vi "PC Engine.vi"(2 "Error In":errorcluster) -> (0 "Error Out":errorcluster, 1 "InvalidResponses":string)   [LabVIEW 2013]
uses:
  State Ctrl (PC).ctl
  <vilib>/NI/STM/TCP/TCP Connection Info.ctl
  <vilib>/NI/STM/SubVIs/MetaDataElement.ctl
  Event Mode.ctl
  <vilib>/NI/STM/TCP/TCP Read Options.ctl
  RT/RTsend PCrecv CMD.ctl
  TypeDef/ConnSettingCluster.ctl
  <vilib>/NI/STM/TCP/Read Meta Data (TCP Ref).vi
  <vilib>/NI/STM/TCP/Read Message (TCP).vi
  <vilib>/NI/STM/TCP/Read Meta Data (TCP Clst).vi
  <vilib>/NI/STM/TCP/Write Message (TCP).vi
  <vilib>/NI/STM/NI STM.lvlib
panel:
  out "Send Conn Info":T1
  in  "State Control":T3
  in  "Recv Port":u16=5555
  in  "Stop":bool
  out "Connected?":bool
  in  "ConnectAttemptLimit":u32=5
  in  "Send Port":u16=5555
  in  "RIO IP Address":string
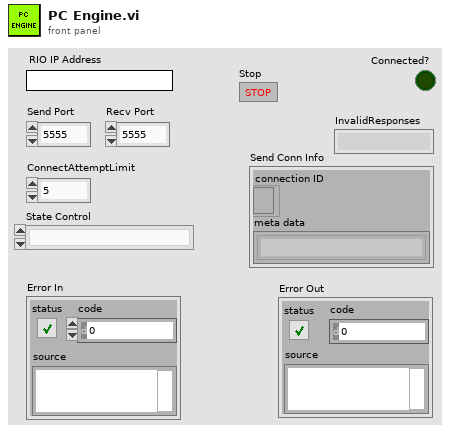
[diagram p1: front panel]
types:
  T1 = typedef "NI STM.lvlib/TCP Connection Info.ctl" = cluster{"connection ID":refnum<k5>, "meta data":T2[]}
  T2 = typedef "NI STM.lvlib/MetaDataElement.ctl" = string
  T3 = typedef "State Ctrl (PC).ctl" = enum16{"", "Send Connect", "Send Connect 2", "Recv Connect", "Recv Connect 2", "No Connection", "Disconnect"}
  T4 = typedef "Event Mode.ctl" = enum16{"Init", "Get", "Set", "Destroy"}
  T5 = cluster{"Command":string, "Flattened Data":string}
  T6 = typedef "PCsend RTrecv CMD.ctl" = enum16{"ConnSettings", "Connect", "Stop", "Digital Outputs", "Analog Outputs", "Sweep Parameters", "Start Sweep", "Cal2RT", "Save Cal", "Load Cal"}
  T7 = typedef "ConnSettingCluster.ctl" = cluster{"ConnectAttemptLimit(5)":u32, "IP Address":string, "Send Port":u16, "Recv Port":u16}
  T8 = typedef "NI STM.lvlib/TCP Read Options.ctl" = cluster{"ignore timeout error":bool, "timeout ms (1000)":i32}
  T9 = typedef "RTsend PCrecv CMD.ctl" = enum16{"Digital Inputs", "Connected?", "Data", "Data 2", "Cal2PC"}
  T10 = cluster{"connection ID":bool, "meta data":bool[]}
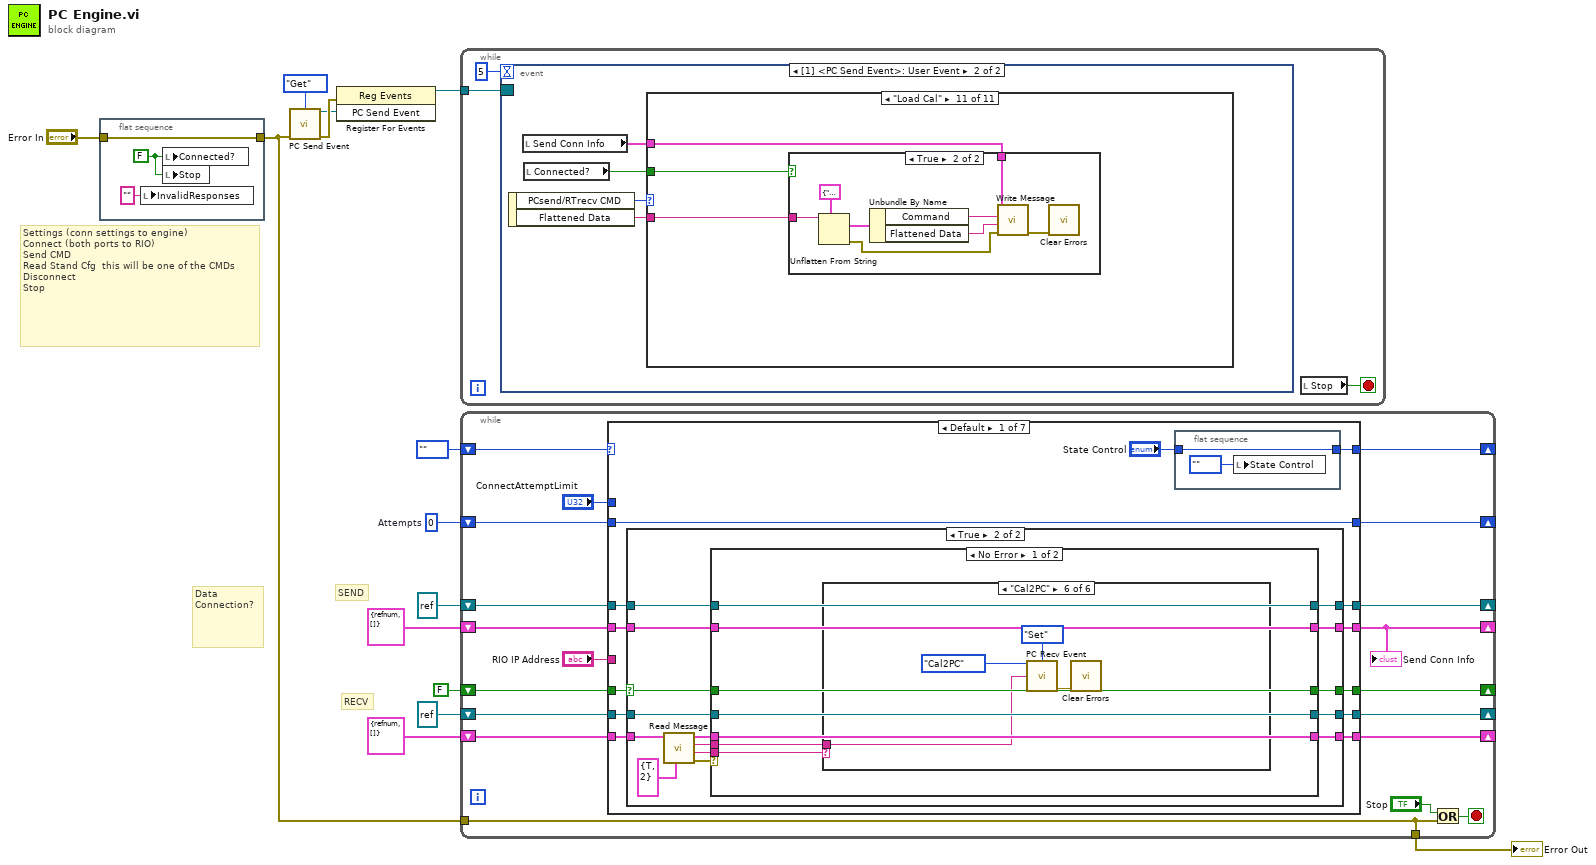
[diagram p0: block diagram]
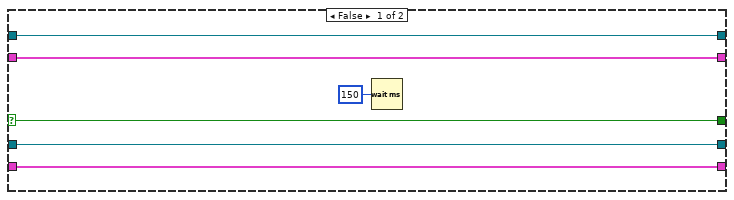
[diagram p2: hidden frame]
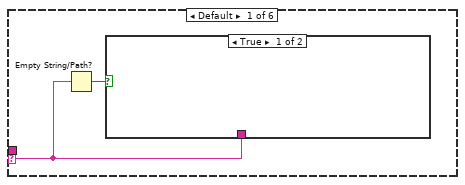
[diagram p3: hidden frame]
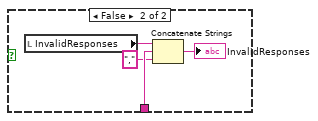
[diagram p4: hidden frame]
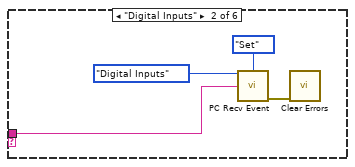
[diagram p5: hidden frame]
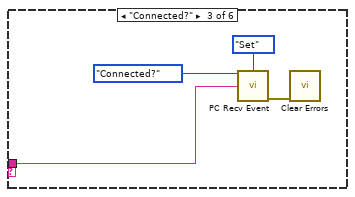
[diagram p6: hidden frame]
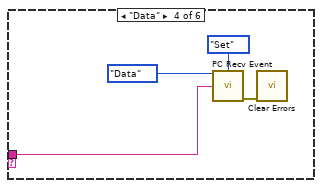
[diagram p7: hidden frame]
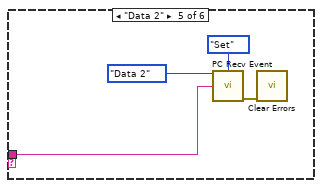
[diagram p8: hidden frame]
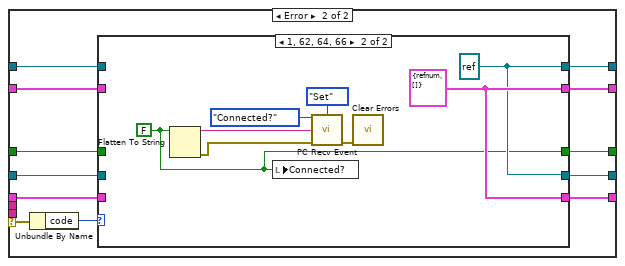
[diagram p9: hidden frame]
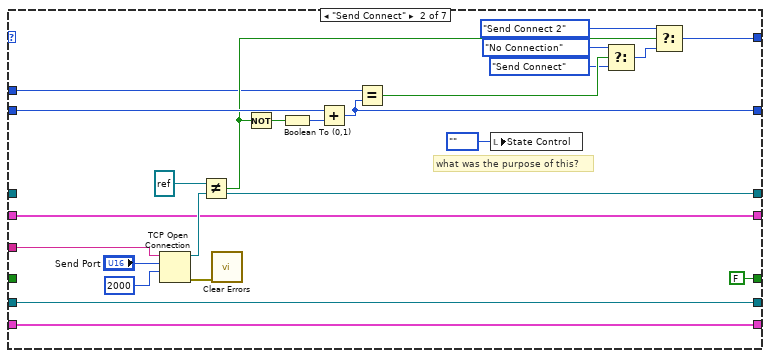
[diagram p11: hidden frame]
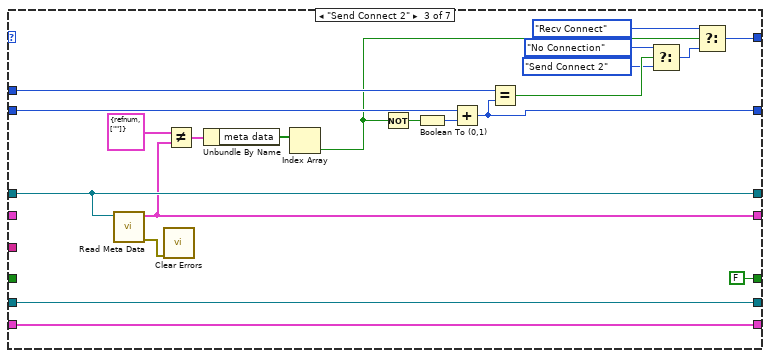
[diagram p12: hidden frame]
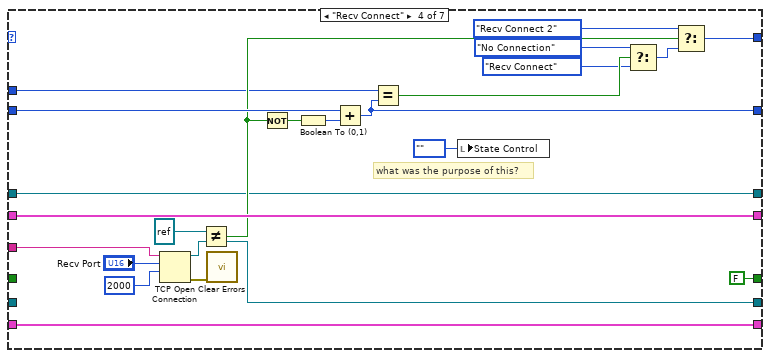
[diagram p13: hidden frame]
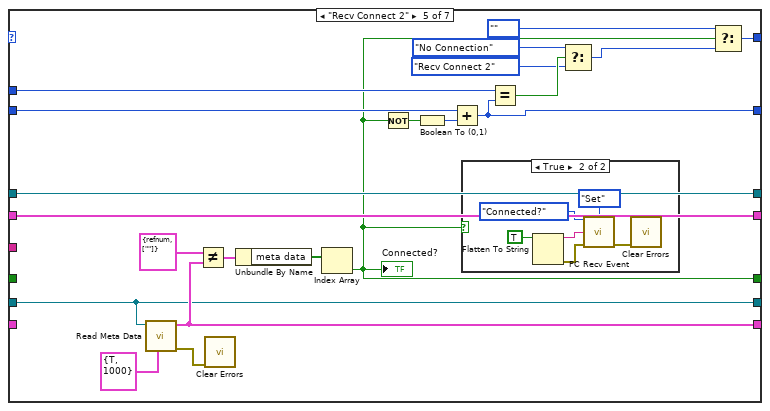
[diagram p14: hidden frame]
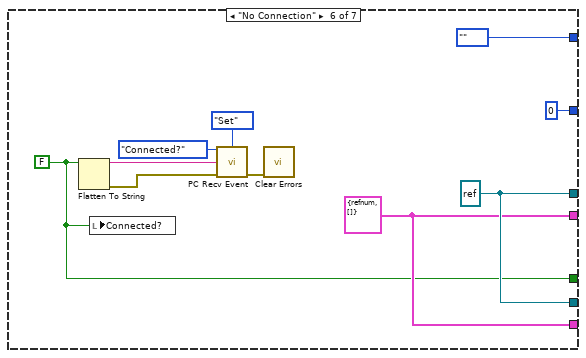
[diagram p16: hidden frame]
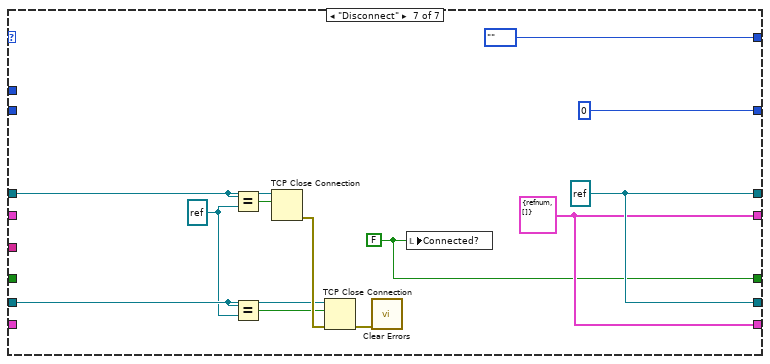
[diagram p17: hidden frame]
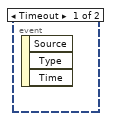
[diagram p18: hidden frame]
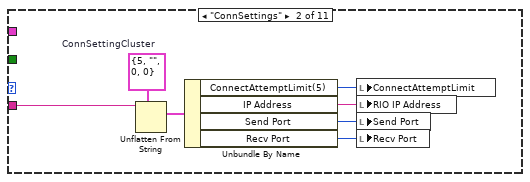
[diagram p20: hidden frame]
diagram:
  w12 = u32 0  # Attempts
  # "RECV"
  # "SEND"
  # "Data\nConnection?"
  # "Settings (conn settings to engine)\nConnect (both ports to RIO)\nSend CMD\nRead Stand Cfg  this will be one of the CMDs\nDisconnect\nStop"
  n1 = flat-sequence {
    tunnel: "Error In" -> [w16]
    tunnel: [w16] -> w10
    frame #0 {
      w17 = FALSE ("Connected?")
      n2 = local write "InvalidResponses"("" ("InvalidResponse")) -> ()
      n3 = local write "Connected?"(w17) -> ()
      n4 = local write "Stop"(w17) -> ()
    }
  }
  n5 = call "PC Send Event.vi"("Mode"=Event_Mode."Get", "Error In"=w10) -> ("PC Send Event"=w5:refnum<user-event>, "Error Out"=w7:errorcluster)  [unwired: 12 in]
  n6 = register-events(error in=w7, w5) -> (reference out=w6:refnum<event-registration>)  [unwired: 1 in, 1 out]
  n7 = while {
    tunnel: w6 -> [w18]
    stop <- w20 stop-if-true
    n8 = event shown="[1] <PC Send Event>: User Event" {
      selector: w18 -> [_ _]
      dyn-events: _ -> [_ _]
      timeout: 5 ("evtime") -> [_ _]
      event Timeout {
        n9 = event-data() -> ()  [unwired: 1 in, 3 out]
      }
      event User Event {
        n10 = event-data() -> ("PCsend/RTrecv CMD"=w21:T6, "Flattened Data"=w24:string)  [unwired: 1 in]
        n11 = local read "Send Conn Info"() -> (w23:T1)
        n12 = local read "Connected?"() -> (w22:bool)
        n13 = case shown="\"Load Cal\"" w21 {
          tunnel: w24 -> [_ w26 _ w36 w47 w58 w69 w80 w91 w102 w113]
          tunnel: w23 -> [_ _ _ w34 w45 w56 w67 w78 w89 w100 w111]
          tunnel: w22 -> [_ _ _ w35 w46 w57 w68 w79 w90 w101 w112]
          frame Default {
          }
          frame "ConnSettings" {
            w25 = T7 {"ConnectAttemptLimit(5)"=5, "IP Address"="", "Send Port"=0, "Recv Port"=0}  # ConnSettingCluster
            n14 = Unflatten From String(type=w25, binary string=w26) -> (value=w31:T7)  [unwired: 3 in, 2 out]
            n15 = Unbundle By Name(w31) -> ("ConnectAttemptLimit(5)"=w29:u32, "IP Address"=w28:string, "Send Port"=w30:u16, "Recv Port"=w27:u16)
            n16 = local write "ConnectAttemptLimit"(w29) -> ()
            n17 = local write "RIO IP Address"(w28) -> ()
            n18 = local write "Send Port"(w30) -> ()
            n19 = local write "Recv Port"(w27) -> ()
          }
          frame "Connect" {
            n20 = local write "State Control"(State_Ctrl_(PC)."Send Connect" ("State Control")) -> ()
          }
          frame "Stop" {
            n21 = case shown="True" w35 {
              tunnel: w36 -> [_ w44]
              tunnel: w34 -> [_ w39]
              frame False {
              }
              frame True {
                n22 = Unflatten From String(type=T5 {"Command"="", "Flattened Data"=""} ("cluster"), binary string=w44) -> (value=w43:T5, error out=w37:errorcluster)  [unwired: 3 in, 1 out]
                n23 = Unbundle By Name(w43) -> ("Command"=w40:string, "Flattened Data"=w41:string)
                n24 = call-poly <vilib>:"Write Message.vi"("error in"=w37, "data"=w41, "name"=w40, "connection info in"=w39) -> ("error out"=w38:errorcluster)  [unwired: 6 in, 1 out]
                n25 = call <vilib>:"Clear Errors.vi"("error in (no error)"=w38) -> ()  [unwired: 6 in, 1 out]
              }
            }
            n26 = local write "Stop"(TRUE ("Stop")) -> ()
          }
          frame "Digital Outputs" {
            n27 = case shown="False" w46 {
              tunnel: w47 -> [_ w55]
              tunnel: w45 -> [_ w50]
              frame False {
              }
              frame True {
                n28 = Unflatten From String(type=T5 {"Command"="", "Flattened Data"=""} ("cluster"), binary string=w55) -> (value=w54:T5, error out=w48:errorcluster)  [unwired: 3 in, 1 out]
                n29 = Unbundle By Name(w54) -> ("Command"=w51:string, "Flattened Data"=w52:string)
                n30 = call-poly <vilib>:"Write Message.vi"("error in"=w48, "data"=w52, "name"=w51, "connection info in"=w50) -> ("error out"=w49:errorcluster)  [unwired: 6 in, 1 out]
                n31 = call <vilib>:"Clear Errors.vi"("error in (no error)"=w49) -> ()  [unwired: 6 in, 1 out]
              }
            }
          }
          frame "Analog Outputs" {
            n32 = case shown="True" w57 {
              tunnel: w58 -> [_ w66]
              tunnel: w56 -> [_ w61]
              frame False {
              }
              frame True {
                n33 = Unflatten From String(type=T5 {"Command"="", "Flattened Data"=""} ("cluster"), binary string=w66) -> (value=w65:T5, error out=w59:errorcluster)  [unwired: 3 in, 1 out]
                n34 = Unbundle By Name(w65) -> ("Command"=w62:string, "Flattened Data"=w63:string)
                n35 = call-poly <vilib>:"Write Message.vi"("error in"=w59, "data"=w63, "name"=w62, "connection info in"=w61) -> ("error out"=w60:errorcluster)  [unwired: 6 in, 1 out]
                n36 = call <vilib>:"Clear Errors.vi"("error in (no error)"=w60) -> ()  [unwired: 6 in, 1 out]
              }
            }
          }
          frame "Sweep Parameters" {
            n37 = case shown="True" w68 {
              tunnel: w69 -> [_ w77]
              tunnel: w67 -> [_ w72]
              frame False {
              }
              frame True {
                n38 = Unflatten From String(type=T5 {"Command"="", "Flattened Data"=""} ("cluster"), binary string=w77) -> (value=w76:T5, error out=w70:errorcluster)  [unwired: 3 in, 1 out]
                n39 = Unbundle By Name(w76) -> ("Command"=w73:string, "Flattened Data"=w74:string)
                n40 = call-poly <vilib>:"Write Message.vi"("error in"=w70, "data"=w74, "name"=w73, "connection info in"=w72) -> ("error out"=w71:errorcluster)  [unwired: 6 in, 1 out]
                n41 = call <vilib>:"Clear Errors.vi"("error in (no error)"=w71) -> ()  [unwired: 6 in, 1 out]
              }
            }
          }
          frame "Start Sweep" {
            n42 = case shown="True" w79 {
              tunnel: w80 -> [_ w88]
              tunnel: w78 -> [_ w83]
              frame False {
              }
              frame True {
                n43 = Unflatten From String(type=T5 {"Command"="", "Flattened Data"=""} ("cluster"), binary string=w88) -> (value=w87:T5, error out=w81:errorcluster)  [unwired: 3 in, 1 out]
                n44 = Unbundle By Name(w87) -> ("Command"=w84:string, "Flattened Data"=w85:string)
                n45 = call-poly <vilib>:"Write Message.vi"("error in"=w81, "data"=w85, "name"=w84, "connection info in"=w83) -> ("error out"=w82:errorcluster)  [unwired: 6 in, 1 out]
                n46 = call <vilib>:"Clear Errors.vi"("error in (no error)"=w82) -> ()  [unwired: 6 in, 1 out]
              }
            }
          }
          frame "Cal2RT" {
            n47 = case shown="True" w90 {
              tunnel: w91 -> [_ w99]
              tunnel: w89 -> [_ w94]
              frame False {
              }
              frame True {
                n48 = Unflatten From String(type=T5 {"Command"="", "Flattened Data"=""} ("cluster"), binary string=w99) -> (value=w98:T5, error out=w92:errorcluster)  [unwired: 3 in, 1 out]
                n49 = Unbundle By Name(w98) -> ("Command"=w95:string, "Flattened Data"=w96:string)
                n50 = call-poly <vilib>:"Write Message.vi"("error in"=w92, "data"=w96, "name"=w95, "connection info in"=w94) -> ("error out"=w93:errorcluster)  [unwired: 6 in, 1 out]
                n51 = call <vilib>:"Clear Errors.vi"("error in (no error)"=w93) -> ()  [unwired: 6 in, 1 out]
              }
            }
          }
          frame "Save Cal" {
            n52 = case shown="True" w101 {
              tunnel: w102 -> [_ w110]
              tunnel: w100 -> [_ w105]
              frame False {
              }
              frame True {
                n53 = Unflatten From String(type=T5 {"Command"="", "Flattened Data"=""} ("cluster"), binary string=w110) -> (value=w109:T5, error out=w103:errorcluster)  [unwired: 3 in, 1 out]
                n54 = Unbundle By Name(w109) -> ("Command"=w106:string, "Flattened Data"=w107:string)
                n55 = call-poly <vilib>:"Write Message.vi"("error in"=w103, "data"=w107, "name"=w106, "connection info in"=w105) -> ("error out"=w104:errorcluster)  [unwired: 6 in, 1 out]
                n56 = call <vilib>:"Clear Errors.vi"("error in (no error)"=w104) -> ()  [unwired: 6 in, 1 out]
              }
            }
          }
          frame "Load Cal" {
            n57 = case shown="True" w112 {
              tunnel: w113 -> [_ w121]
              tunnel: w111 -> [_ w116]
              frame False {
              }
              frame True {
                n58 = Unflatten From String(type=T5 {"Command"="", "Flattened Data"=""} ("cluster"), binary string=w121) -> (value=w120:T5, error out=w114:errorcluster)  [unwired: 3 in, 1 out]
                n59 = Unbundle By Name(w120) -> ("Command"=w117:string, "Flattened Data"=w118:string)
                n60 = call-poly <vilib>:"Write Message.vi"("error in"=w114, "data"=w118, "name"=w117, "connection info in"=w116) -> ("error out"=w115:errorcluster)  [unwired: 6 in, 1 out]
                n61 = call <vilib>:"Clear Errors.vi"("error in (no error)"=w115) -> ()  [unwired: 6 in, 1 out]
              }
            }
          }
        }
      }
    }
    n62 = local read "Stop"() -> (w20:bool)
  }
  n63 = while {
    shift-right: [w135] -> _
    shift-left: refnum<k5> refnum ("connection ID") -> [w138]
    shift-right: [w136] -> _
    shift-left: T1 {"connection ID"=refnum, "meta data"=[]} ("connection info out") -> [w137]
    shift-right: [w139] -> _
    shift-left: State_Ctrl_(PC)."" ("State Control") -> [w140]
    shift-right: [w133] -> _
    shift-left: w12 -> [w134]
    tunnel: w10 -> [w122]
    shift-right: [w126] -> _
    shift-left: refnum<k5> refnum ("connection ID") -> [w128]
    shift-right: [w125] -> _
    shift-left: T1 {"connection ID"=refnum, "meta data"=[]} ("connection info out") -> [w127]
    shift-right: [w123] -> _
    shift-left: FALSE -> [w124]
    tunnel: [w122] -> w1
    stop <- w131 stop-if-true
    n64 = case shown="Default" w140 {
      tunnel: [w153 w257 w275 w301 w319 State_Ctrl_(PC)."" ("State Control") State_Ctrl_(PC)."" ("State Control")] -> w139
      tunnel: w138 -> [w148 _ w276 w283 w320 _ w345]
      tunnel: w137 -> [w149 w252 _ w298 w307 _ _]
      tunnel: [w145 w252 w259 w298 w307 w333 w347] -> w136
      tunnel: [w146 w253 w276 w283 w320 w334 w348] -> w135
      tunnel: w134 -> [w141 w251 w271 w297 w315 _ _]
      tunnel: [w141 w247 w270 w293 w314 u32 0 ("Attempts") u32 0 ("Attempts")] -> w133
      tunnel: "ConnectAttemptLimit" -> [_ w244 w268 w290 w312 _ _]
      tunnel: "RIO IP Address" -> [_ w239 _ w285 _ _ _]
      tunnel: w128 -> [w147 w238 w264 _ w306 _ w342]
      tunnel: w127 -> [w150 w237 w263 w281 _ _ _]
      tunnel: [w143 w238 w264 w282 w306 w334 w348] -> w126
      tunnel: [w142 w237 w263 w281 w308 w333 w347] -> w125
      tunnel: w124 -> [w151 _ _ _ _ _ _]
      tunnel: [w144 FALSE ("Meta Element") FALSE ("Meta Element") FALSE ("Meta Element") w303 w332 w340] -> w123
      frame Default {
        n65 = case shown="True" w151 {
          selector: w151 -> [w157 w168]
          tunnel: w150 -> [w155 w173]
          tunnel: w149 -> [w158 w169]
          tunnel: w148 -> [w159 w167]
          tunnel: w147 -> [w156 w170]
          tunnel: [w159 w165] -> w146
          tunnel: [w158 w163] -> w145
          tunnel: [w157 w166] -> w144
          tunnel: [w156 w164] -> w143
          tunnel: [w155 w162] -> w142
          frame False {
            n66 = Wait (ms)(milliseconds to wait=u32 150) -> ()  [unwired: 1 out]
          }
          frame True {
            n67 = call-poly <vilib>:"Read Message.vi"("options"=T8 {"ignore timeout error"=TRUE, "timeout ms (1000)"=2}, "connection info in"=w173) -> ("error out"=w172:errorcluster, "name"=w161:T2, "data string"=w160:string, "connection info out"=w171:T1)  [unwired: 4 in, 2 out]
            n68 = case shown="No Error" w172 {
              selector: w172 -> [_ w219]
              tunnel: w171 -> [w177 w217]
              tunnel: w170 -> [w178 w216]
              tunnel: w169 -> [w180 w214]
              tunnel: w168 -> [w179 w215]
              tunnel: w167 -> [w181 w213]
              tunnel: [w179 w210] -> w166
              tunnel: [w181 w212] -> w165
              tunnel: [w178 w209] -> w164
              tunnel: [w180 w211] -> w163
              tunnel: [w177 w208] -> w162
              tunnel: w161 -> [w176 _]
              tunnel: w160 -> [w175 _]
              frame No Error {
                n69 = case shown="\"Cal2PC\"" w176 {
                  selector: w176 -> [w183 _ _ _ _ _]
                  tunnel: w175 -> [_ w188 w194 w199 w203 w207]
                  frame Default {
                    n70 = Empty String/Path?(string/path=w183) -> (empty?=w182:bool)
                    n71 = case shown="True" w182 {
                      tunnel: w183 -> [_ w186]
                      frame True {
                      }
                      frame False {
                        n72 = local read "InvalidResponses"() -> (w187:string)
                        n73 = Concatenate Strings(w187, w186, "," ("string")) -> (→"InvalidResponses":string)
                      }
                    }
                  }
                  frame "Digital Inputs" {
                    n74 = call "PC Recv Event.vi"("RTsend/PCrecv CMD"=RTsend_PCrecv_CMD."Digital Inputs", "Mode"=Event_Mode."Set", "Flattened Data"=w188) -> ("Error Out"=w190:errorcluster)  [unwired: 11 in, 1 out]
                    n75 = call <vilib>:"Clear Errors.vi"("error in (no error)"=w190) -> ()  [unwired: 6 in, 1 out]
                  }
                  frame "Connected?" {
                    n76 = call "PC Recv Event.vi"("RTsend/PCrecv CMD"=RTsend_PCrecv_CMD."Connected?", "Mode"=Event_Mode."Set", "Flattened Data"=w194) -> ("Error Out"=w193:errorcluster)  [unwired: 11 in, 1 out]
                    n77 = call <vilib>:"Clear Errors.vi"("error in (no error)"=w193) -> ()  [unwired: 6 in, 1 out]
                  }
                  frame "Data" {
                    n78 = call "PC Recv Event.vi"("RTsend/PCrecv CMD"=RTsend_PCrecv_CMD."Data", "Mode"=Event_Mode."Set", "Flattened Data"=w199) -> ("Error Out"=w197:errorcluster)  [unwired: 11 in, 1 out]
                    n79 = call <vilib>:"Clear Errors.vi"("error in (no error)"=w197) -> ()  [unwired: 6 in, 1 out]
                  }
                  frame "Data 2" {
                    n80 = call "PC Recv Event.vi"("RTsend/PCrecv CMD"=RTsend_PCrecv_CMD."Data 2", "Mode"=Event_Mode."Set", "Flattened Data"=w203) -> ("Error Out"=w201:errorcluster)  [unwired: 11 in, 1 out]
                    n81 = call <vilib>:"Clear Errors.vi"("error in (no error)"=w201) -> ()  [unwired: 6 in, 1 out]
                  }
                  frame "Cal2PC" {
                    n82 = call "PC Recv Event.vi"("RTsend/PCrecv CMD"=RTsend_PCrecv_CMD."Cal2PC", "Mode"=Event_Mode."Set", "Flattened Data"=w207) -> ("Error Out"=w205:errorcluster)  [unwired: 11 in, 1 out]
                    n83 = call <vilib>:"Clear Errors.vi"("error in (no error)"=w205) -> ()  [unwired: 6 in, 1 out]
                  }
                }
              }
              frame Error {
                n84 = Unbundle By Name(w219) -> ("code"=w218:i32)
                n85 = case shown="1, 62, 64, 66" w218 {
                  tunnel: w217 -> [w220 _]
                  tunnel: w216 -> [w221 _]
                  tunnel: w215 -> [w222 _]
                  tunnel: w214 -> [w223 _]
                  tunnel: w213 -> [w224 _]
                  tunnel: [w224 w231] -> w212
                  tunnel: [w223 w232] -> w211
                  tunnel: [w222 w228] -> w210
                  tunnel: [w221 w231] -> w209
                  tunnel: [w220 w232] -> w208
                  frame Default {
                  }
                  frame 1, 62, 64, 66 {
                    w228 = FALSE ("Connected?")
                    w232 = T1 {"connection ID"=refnum, "meta data"=[]} ("connection info out")
                    w231 = refnum<k5> refnum ("connection ID")
                    n86 = Flatten To String(anything=w228) -> (data string=w229:string, error out=w227:errorcluster)  [unwired: 3 in, 1 out]
                    n87 = local write "Connected?"(w228) -> ()
                    n88 = call "PC Recv Event.vi"("RTsend/PCrecv CMD"=RTsend_PCrecv_CMD."Connected?", "Mode"=Event_Mode."Set", "Flattened Data"=w229, "Error In"=w227) -> ("Error Out"=w226:errorcluster)  [unwired: 10 in, 1 out]
                    n89 = call <vilib>:"Clear Errors.vi"("error in (no error)"=w226) -> ()  [unwired: 6 in, 1 out]
                  }
                }
              }
            }
          }
        }
        n90 = flat-sequence {
          tunnel: "State Control" -> [w234]
          tunnel: [w234] -> w153
          frame #0 {
            n91 = local write "State Control"(State_Ctrl_(PC)."" ("State Control")) -> ()
          }
        }
      }
      frame "Send Connect" {
        # "what was the purpose of this?"
        n92 = TCP Open Connection(address=w239, remote port or service name="Send Port", timeout ms (60000)=2000) -> (connection ID=w253:refnum<k5>, error out=w235:errorcluster)  [unwired: 2 in]
        n93 = Not Equal?(x=refnum<k5> refnum ("connection ID"), y=w253) -> (x != y?=w250:bool)
        n94 = call <vilib>:"Clear Errors.vi"("error in (no error)"=w235) -> ()  [unwired: 6 in, 1 out]
        n95 = Not(x=w250) -> (.not. x?=w249:bool)
        n96 = Boolean To (0,1)(Boolean=w249) -> (0, 1=w248:i16)
        n97 = Add(x=w251, y=w248) -> (x+y=w247:u32)
        n98 = Equal?(x=w244, y=w247) -> (x = y?=w246:bool)
        n99 = local write "State Control"(State_Ctrl_(PC)."" ("State Control")) -> ()
        n100 = Select(t=State_Ctrl_(PC)."No Connection" ("State Control"), s=w246, f=State_Ctrl_(PC)."Send Connect" ("State Control")) -> (s? t:f=w245:T3)
        n101 = Select(t=State_Ctrl_(PC)."Send Connect 2" ("State Control"), s=w250, f=w245) -> (s? t:f=w257:T3)
      }
      frame "Send Connect 2" {
        n102 = call-poly <vilib>:"Read Meta Data.vi"("connection ID"=w276) -> ("error out"=w260:errorcluster, "connection info out"=w259:T1)  [unwired: 8 in, 1 out]
        n103 = call <vilib>:"Clear Errors.vi"("error in (no error)"=w260) -> ()  [unwired: 6 in, 1 out]
        n104 = Not Equal?(x=T1 {"connection ID"=refnum, "meta data"=[""]} ("connection info out"), y=w259) -> (x != y?=w278:T10)
        n105 = Unbundle By Name(w278) -> ("meta data"=w267:bool[])
        n106 = Index Array(array=w267) -> (element=w258:bool)  [unwired: 1 in]
        n107 = Not(x=w258) -> (.not. x?=w273:bool)
        n108 = Boolean To (0,1)(Boolean=w273) -> (0, 1=w272:i16)
        n109 = Add(x=w271, y=w272) -> (x+y=w270:u32)
        n110 = Equal?(x=w268, y=w270) -> (x = y?=w269:bool)
        n111 = Select(t=State_Ctrl_(PC)."No Connection" ("State Control"), s=w269, f=State_Ctrl_(PC)."Send Connect 2" ("State Control")) -> (s? t:f=w274:T3)
        n112 = Select(t=State_Ctrl_(PC)."Recv Connect" ("State Control"), s=w258, f=w274) -> (s? t:f=w275:T3)
      }
      frame "Recv Connect" {
        # "what was the purpose of this?"
        n113 = TCP Open Connection(address=w285, remote port or service name="Recv Port", timeout ms (60000)=2000) -> (connection ID=w282:refnum<k5>, error out=w279:errorcluster)  [unwired: 2 in]
        n114 = Not Equal?(x=refnum<k5> refnum ("connection ID"), y=w282) -> (x != y?=w296:bool)
        n115 = call <vilib>:"Clear Errors.vi"("error in (no error)"=w279) -> ()  [unwired: 6 in, 1 out]
        n116 = Not(x=w296) -> (.not. x?=w295:bool)
        n117 = Boolean To (0,1)(Boolean=w295) -> (0, 1=w294:i16)
        n118 = Add(x=w297, y=w294) -> (x+y=w293:u32)
        n119 = Equal?(x=w290, y=w293) -> (x = y?=w292:bool)
        n120 = local write "State Control"(State_Ctrl_(PC)."" ("State Control")) -> ()
        n121 = Select(t=State_Ctrl_(PC)."No Connection" ("State Control"), s=w292, f=State_Ctrl_(PC)."Recv Connect" ("State Control")) -> (s? t:f=w291:T3)
        n122 = Select(t=State_Ctrl_(PC)."Recv Connect 2" ("State Control"), s=w296, f=w291) -> (s? t:f=w301:T3)
      }
      frame "Recv Connect 2" {
        n123 = call-poly <vilib>:"Read Meta Data.vi"("options"=T8 {"ignore timeout error"=TRUE, "timeout ms (1000)"=1000}, "connection ID"=w306) -> ("error out"=w305:errorcluster, "connection info out"=w308:T1)  [unwired: 7 in, 1 out]
        n124 = Not Equal?(x=T1 {"connection ID"=refnum, "meta data"=[""]} ("connection info out"), y=w308) -> (x != y?=w322:T10)
        n125 = call <vilib>:"Clear Errors.vi"("error in (no error)"=w305) -> ()  [unwired: 6 in, 1 out]
        n126 = Unbundle By Name(w322) -> ("meta data"=w311:bool[])
        n127 = Index Array(array=w311) -> (element=w303:bool)  [unwired: 1 in]
        "Connected?" <- w303
        n128 = Not(x=w303) -> (.not. x?=w317:bool)
        n129 = Boolean To (0,1)(Boolean=w317) -> (0, 1=w316:i16)
        n130 = Add(x=w315, y=w316) -> (x+y=w314:u32)
        n131 = case shown="True" w303 {
          frame False {
          }
          frame True {
            n132 = Flatten To String(anything=TRUE) -> (data string=w326:string, error out=w325:errorcluster)  [unwired: 3 in, 1 out]
            n133 = call "PC Recv Event.vi"("RTsend/PCrecv CMD"=RTsend_PCrecv_CMD."Connected?", "Mode"=Event_Mode."Set", "Flattened Data"=w326, "Error In"=w325) -> ("Error Out"=w324:errorcluster)  [unwired: 10 in, 1 out]
            n134 = call <vilib>:"Clear Errors.vi"("error in (no error)"=w324) -> ()  [unwired: 6 in, 1 out]
          }
        }
        n135 = Equal?(x=w312, y=w314) -> (x = y?=w313:bool)
        n136 = Select(t=State_Ctrl_(PC)."No Connection" ("State Control"), s=w313, f=State_Ctrl_(PC)."Recv Connect 2" ("State Control")) -> (s? t:f=w318:T3)
        n137 = Select(t=State_Ctrl_(PC)."" ("State Control"), s=w303, f=w318) -> (s? t:f=w319:T3)
      }
      frame "No Connection" {
        w332 = FALSE
        w333 = T1 {"connection ID"=refnum, "meta data"=[]} ("connection info out")
        w334 = refnum<k5> refnum ("connection ID")
        n138 = Flatten To String(anything=w332) -> (data string=w336:string, error out=w331:errorcluster)  [unwired: 3 in, 1 out]
        n139 = local write "Connected?"(w332) -> ()
        n140 = call "PC Recv Event.vi"("RTsend/PCrecv CMD"=RTsend_PCrecv_CMD."Connected?", "Mode"=Event_Mode."Set", "Flattened Data"=w336, "Error In"=w331) -> ("Error Out"=w330:errorcluster)  [unwired: 10 in, 1 out]
        n141 = call <vilib>:"Clear Errors.vi"("error in (no error)"=w330) -> ()  [unwired: 6 in, 1 out]
      }
      frame "Disconnect" {
        w340 = FALSE ("Connected?")
        w341 = refnum<k5> refnum ("connection ID")
        w347 = T1 {"connection ID"=refnum, "meta data"=[]} ("connection info out")
        w348 = refnum<k5> refnum ("connection ID")
        n142 = Equal?(x=w345, y=w341) -> (x = y?=w344:bool)
        n143 = Equal?(x=w342, y=w341) -> (x = y?=w343:bool)
        n144 = TCP Close Connection(connection ID=w345, abort (F)=w344) -> (error out=w346:errorcluster)  [unwired: 1 in, 1 out]
        n145 = TCP Close Connection(connection ID=w342, abort (F)=w343, error in (no error)=w346) -> (error out=w339:errorcluster)  [unwired: 1 out]
        n146 = call <vilib>:"Clear Errors.vi"("error in (no error)"=w339) -> ()  [unwired: 6 in, 1 out]
        n147 = local write "Connected?"(w340) -> ()
      }
    }
    "Send Conn Info" <- w136
    n148 = Or(x="Stop", y=w122) -> (x .or. y?=w131:bool)
  }
  "Error Out" <- w1
